vi "FSMPos_GetMeasurement_Test.vi"(3 "output control":T1, 4 "data":T2, 5 "X":dbl[](array[numeric])) -> (0 "error out":errorcluster, 1 "gradient":dbl[](array[numeric]), 2 "f(X)":dbl)   [LabVIEW 2019]
uses:
  <vilib>/gmath/NumericalOptimization/objective function data.ctl
  <vilib>/gmath/NI_Gmath.lvlib
panel:
  out "Cursor Y":dbl
  out "Cursor X":dbl
  out "Array":dbl[][](array[numeric])
  out "Yindex":dbl
  out "XY Intensity Map 2":dbl[][](graph) caption="XY Intensity Map"
  out "element":dbl
  out "Xindex":dbl
  out "XY Intensity Map":dbl[][](graph)
  # "Input"
  # "Output"
  # "Indices in 2D array and value"
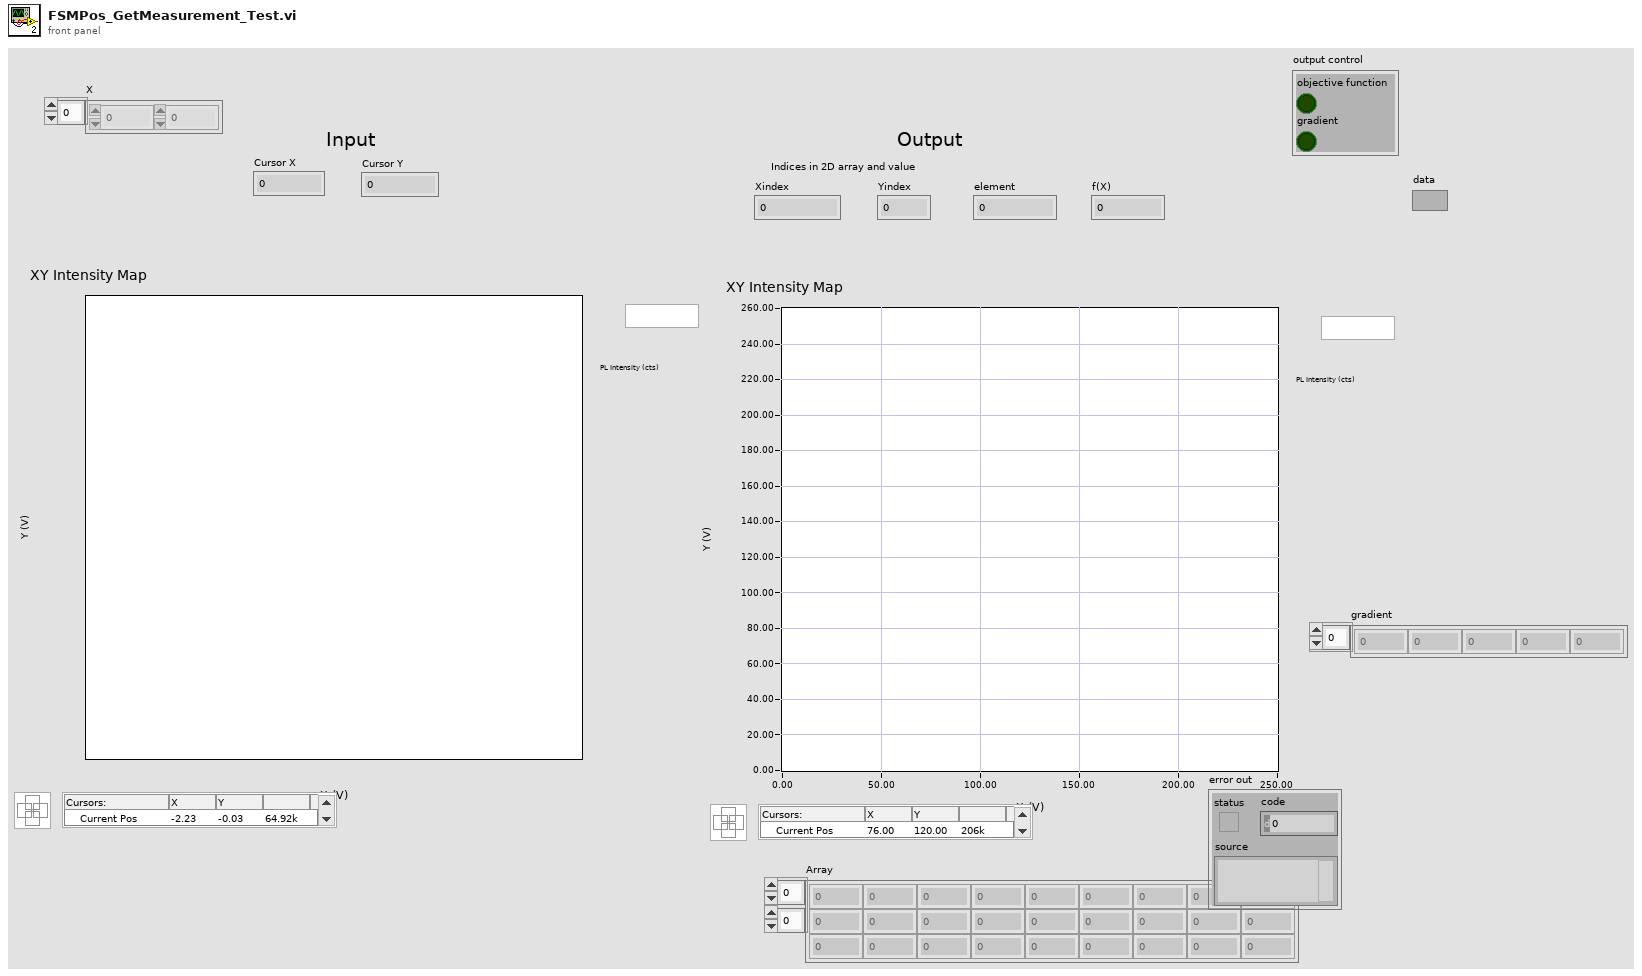
[diagram p1: front panel]
types:
  T1 = cluster{"objective function":bool, "gradient":bool}
  T2 = typedef "NI_Gmath.lvlib/objective function data.ctl" = variant
  T3 = typedef "LVPointDoubleTypeDef.ctl" = cluster{"Cursor X":dbl, "Cursor Y":dbl}
  T4 = typedef "LVOffsetAndMultiplierTypeDef.ctl" = cluster{"Offset":dbl, "Multiplier":dbl}
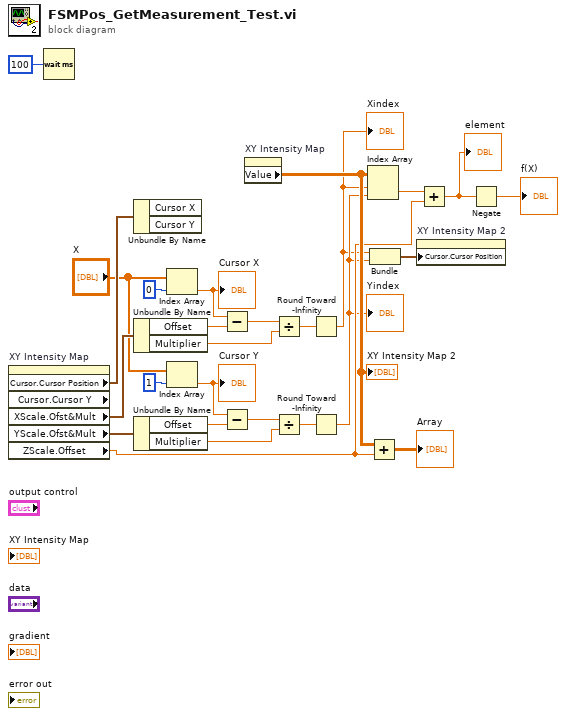
[diagram p0: block diagram]
diagram:
  n1 = property on="XY Intensity Map" class="IntGraph (strict)" props=["Cursor", "Cursor Position", "Cursor", "Cursor Y", "XScale", "Ofst&Mult", "YScale", "Ofst&Mult", "ZScale", "Offset"]() -> ("Cursor.Cursor Position"=w25:T3, "XScale.Ofst&Mult"=w26:T4, "YScale.Ofst&Mult"=w22:T4, "ZScale.Offset"=w12:dbl)  [unwired: 2 in, 3 out]
  n2 = Wait (ms)(milliseconds to wait=u32 100) -> ()  [unwired: 1 out]
  n3 = Unbundle By Name(w25) -> ()  [unwired: 2 out]
  n4 = Unbundle By Name(w26) -> ("Offset"=w24:dbl, "Multiplier"=w23:dbl)
  n5 = Unbundle By Name(w22) -> ("Offset"=w20:dbl, "Multiplier"=w21:dbl)
  n6 = Index Array(array="X", index=0) -> (element=w3:dbl)
  "Cursor X" <- w3
  n7 = Index Array(array="X", index=1) -> (element=w2:dbl)
  "Cursor Y" <- w2
  n8 = Subtract(x=w3, y=w24) -> (x-y=w15:dbl)
  n9 = Subtract(x=w2, y=w20) -> (x-y=w17:dbl)
  n10 = property on="XY Intensity Map" class="IntGraph (strict)"() -> ("Value"=w13:dbl[][])  [unwired: 2 in, 2 out]
  "XY Intensity Map 2" <- w13
  n11 = Divide(x=w15, y=w23) -> (x/y=w14:dbl)
  n12 = Divide(x=w17, y=w21) -> (x/y=w19:dbl)
  n13 = Round Toward -Infinity(1:w14) -> (0:w10:dbl)
  "Xindex" <- w10
  n14 = Round Toward -Infinity(1:w19) -> (0:w11:dbl)
  "Yindex" <- w11
  n15 = Index Array(array=w13, index (row)=w10, index (col)=w11) -> (element=w18:dbl)
  n16 = Add(x=w13, y=w12) -> (x+y=→"Array":dbl[][])
  n17 = Bundle(w10, w11) -> (w16:cluster{dbl, dbl})  [unwired: 1 in]
  n18 = property on="XY Intensity Map 2" class="IntGraph (strict)"("Cursor.Cursor Position"=w16) -> ()  [unwired: 2 in, 2 out]
  n19 = Add(x=w18, y=w12) -> (x+y=w8:dbl)
  "element" <- w8
  n20 = Negate(x=w8) -> (-x=→"f(X)":dbl)
